vi "Write State.vi"(8 "error in (no error)":errorcluster, 10 "State":string, 11 "State Machine in":refnum<class "CCS_State Machine.lvclass">) -> (0 "error out":errorcluster, 3 "State Machine out":refnum<class "CCS_State Machine.lvclass">)   [LabVIEW 2018, in "CCS_State Machine.lvclass"]
uses:
  CCS_State Machine.lvclass
  CCS_State Machine.lvclass/CCS_State Machine.ctl
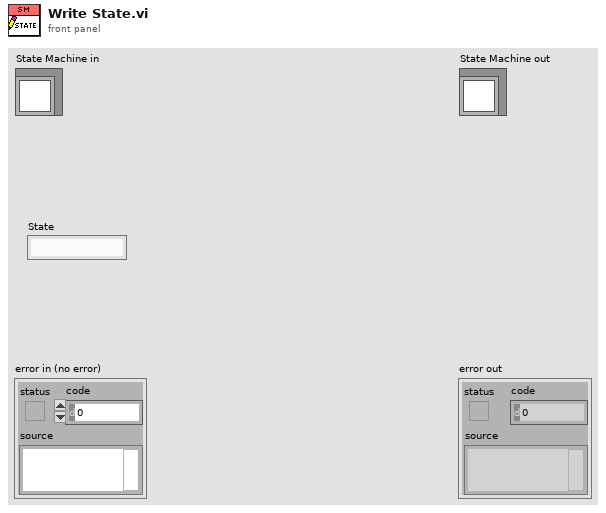
[diagram p1: front panel]
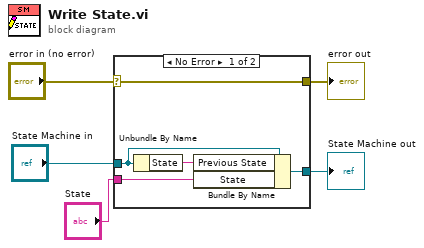
[diagram p0: block diagram]
diagram:
  n1 = case shown="No Error" "error in (no error)" {
    selector: "error in (no error)" -> [w10 w11]
    tunnel: [w10 w11] -> w4
    tunnel: [w9 w12] -> w2
    tunnel: "State Machine in" -> [w7 w12]
    tunnel: "State" -> [w8 _]
    frame No Error {
      n2 = Unbundle By Name(w7) -> ("State"=w6:string)
      n3 = Bundle By Name(cluster=w7, "Previous State"=w6, "State"=w8) -> (w9:refnum<class "CCS_State Machine.lvclass">)
    }
    frame Error {
    }
  }
  "error out" <- w4
  "State Machine out" <- w2
